vi "oa_Truncate Revolution Indices.vi"(6 "last indices":dbl format="%.2f", 7 "reset? (True)":bool=TRUE, 8 "spectral settings":T2={"window type"=1, "number of lines"=400} {"number of lines" min=2; "window type" items=["None"=0, "Hanning"=1, "Hamming"=2, "Blackman-Harris"=3, "Exact Blackman"=4, "Blackman"=5, "Flat Top"=6, "4 Term B-Harris"=7, "7 Term B-Harris"=8, "Low Sidelobe"=9, "Gaussian"=62]}, 9 "X scale in":cluster{"offset":dbl, "multiplier":dbl} {"multiplier" format="%.2f"; "offset" format="%.2f"}, 10 "rev in":dbl[](array[numeric])=[17.400000000000002, 17.6] format="%.2f", 11 "even-angle signal":cluster{"r0":dbl, "dr":dbl, "Y":dbl[]}={"r0"=0.0, "dr"=1.0, "Y"=[]} {"r0" format="%.2p"; "dr" format="%.2p"; "Y" format="%.2f"}) -> (0 "finished":bool, 1 "scales":T1 {"Y scale"."multiplier" format="%.2f"; "Y scale"."offset" format="%.2f"; "X scale"."multiplier" format="%.2f"; "X scale"."offset" format="%.2f"}, 2 "window indices":dbl[](array[numeric]), 3 "data out":dbl[](array[numeric]) format="%.2f")   [LabVIEW 2017, in "SoundVib_Resampling.lvlib"]
uses:
  <vilib>/addons/Sound and Vibration/Order Analysis/Resample Order Tracking/SoundVib_Resampling.lvlib
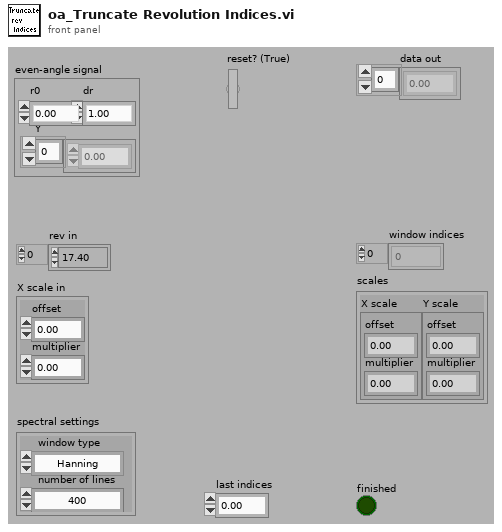
[diagram p1: front panel]
types:
  T1 = cluster{"X scale":cluster{"offset":dbl, "multiplier":dbl}, "Y scale":cluster{"offset":dbl, "multiplier":dbl}}
  T2 = cluster{"window type":u32, "number of lines":i32}
  T3 = cluster{"X scale in":cluster{"offset":dbl, "multiplier":dbl}, cluster{"x/y":dbl, dbl}}
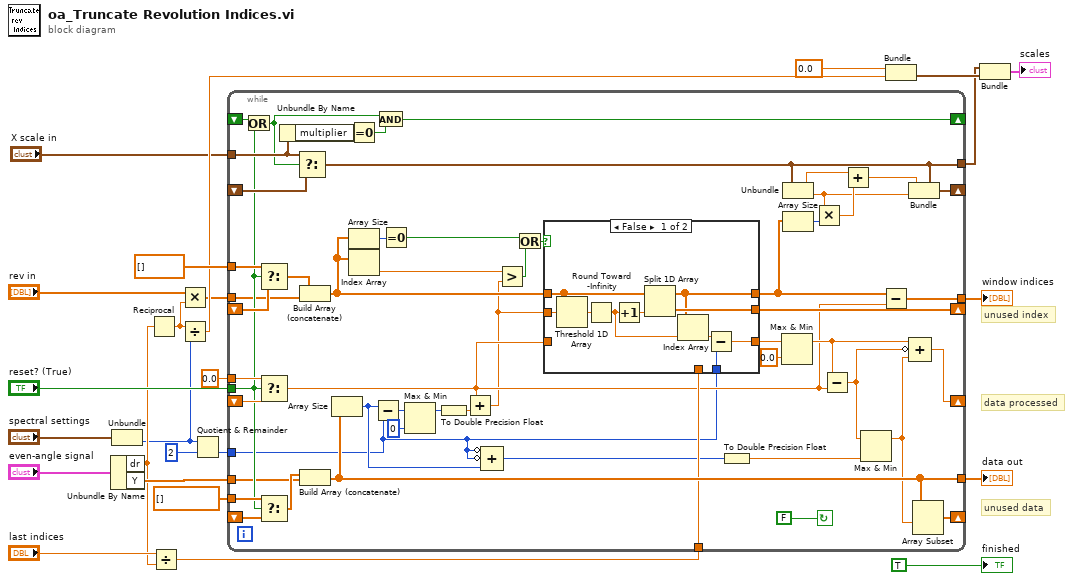
[diagram p0: block diagram]
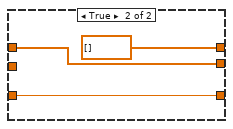
[diagram p2: hidden frame]
diagram:
  # "unused data"
  # "unused index"
  # "data processed"
  n1 = Unbundle By Name("even-angle signal") -> ("dr"=w2:dbl, "Y"=w3:dbl[])
  n2 = Unbundle("spectral settings") -> ("number of lines"=w1:i32)  [unwired: 1 out]
  n3 = Reciprocal(x=w2) -> (1/x=w15:dbl)
  n4 = Divide(x="last indices", y=w2) -> (x/y=w7:dbl)
  n5 = Multiply(x="rev in", y=w15) -> (x*y=w8:dbl[])
  n6 = Divide(x=w15, y=w1) -> (x/y=w14:dbl)
  n7 = Quotient & Remainder(x=w1, y=2) -> (floor(x/y)=w9:i32)  [unwired: 1 out]
  n8 = while {
    shift-right: [w76] -> _
    shift-left: _ -> [w73]
    tunnel: w3 -> [w44]
    shift-right: [w29] -> _
    shift-left: _ -> [w77]
    tunnel: w8 -> [w45]
    tunnel: 0.0 -> [w79]
    shift-right: [w71] -> _
    shift-left: _ -> [w74]
    tunnel: "reset? (True)" -> [w48]
    tunnel: [w70] -> w22
    tunnel: dbl[] [] ("t") -> [w75]
    tunnel: dbl[] [] ("t") -> [w72]
    tunnel: [w67] -> w17
    tunnel: w9 -> [w31]
    tunnel: w7 -> [w60]
    shift-right: [w61] -> _
    shift-left: _ -> [w56]
    tunnel: "X scale in" -> [w53]
    tunnel: [w54] -> w6
    shift-right: [w46] -> _
    shift-left: _ -> [w49]
    stop <- FALSE continue-if-true
    n9 = Or(x=w49, y=w48) -> (x .or. y?=w47:bool)
    n10 = Select(t=w75, s=w48, f=w74) -> (s? t:f=w66:dbl[])
    n11 = Select(t=w79, s=w48, f=w77) -> (s? t:f=w39:dbl)
    n12 = Select(t=w72, s=w48, f=w73) -> (s? t:f=w68:dbl[])
    n13 = Unbundle By Name(w53) -> ("multiplier"=w51:dbl)
    n14 = Select(t=w53, s=w47, f=w56) -> (s? t:f=w54:cluster{"offset":dbl, "multiplier":dbl})
    n15 = Build Array (concatenate)(w66, w45) -> (w38:dbl[])
    n16 = Build Array (concatenate)(w68, w44) -> (w67:dbl[])
    n17 = Array Size(array=w67) -> (size(s)=w32:i32)
    n18 = Equal To 0?(x=w51) -> (x = 0?=w50:bool)
    n19 = Array Size(array=w38) -> (size(s)=w69:i32)
    n20 = Index Array(array=w38) -> (element=w37:dbl)  [unwired: 1 in]
    n21 = Subtract(x=w32, y=w31) -> (x-y=w43:i32)
    n22 = And(x=w47, y=w50) -> (x .and. y?=w46:bool)
    n23 = Equal To 0?(x=w69) -> (x = 0?=w35:bool)
    n24 = Max & Min(x=w43, y=0) -> (max(x,y)=w42:i32)  [unwired: 1 out]
    n25 = To Double Precision Float(number=w42) -> (double precision float=w57:dbl)
    n26 = Add(x=w39, y=w57) -> (x+y=w36:dbl)
    n27 = Compound Arithmetic op=ADD(invert w31, invert w31, w32) -> (w30:i32)
    n28 = Greater?(x=w37, y=w36) -> (0:w34:bool)
    n29 = Or(x=w35, y=w34) -> (x .or. y?=w33:bool)
    n30 = case shown="False" w33 {
      tunnel: w36 -> [w89 _]
      tunnel: [w88 w92] -> w71
      tunnel: w38 -> [w87 w92]
      tunnel: w60 -> [_ _]
      tunnel: [w86 dbl[] []] -> w55
      tunnel: [w85 w90] -> w40
      tunnel: w31 -> [w84 _]
      tunnel: w39 -> [_ w90]
      frame False {
        n31 = Threshold 1D Array(2:w89, 3:w87) -> (0:w83:dbl)  [unwired: 1 in]
        n32 = Round Toward -Infinity(1:w83) -> (0:w82:dbl)
        n33 = Increment(x=w82) -> (x+1=w80:dbl)
        n34 = Split 1D Array(array=w87, index=w80) -> (first subarray=w86:dbl[], second subarray=w88:dbl[])
        n35 = Index Array(array=w86, index=w82) -> (element=w81:dbl)
        n36 = Subtract(x=w81, y=w84) -> (x-y=w85:dbl)
      }
      frame True {
      }
    }
    n37 = To Double Precision Float(number=w30) -> (double precision float=w26:dbl)
    n38 = Max & Min(x=w40, y=0.0) -> (max(x,y)=w58:dbl)  [unwired: 1 out]
    n39 = Unbundle(w54) -> ("offset"=w63:dbl, "multiplier"=w52:dbl)
    n40 = Array Size(array=w55) -> (size(s)=w65:i32)
    n41 = Multiply(x=w52, y=w65) -> (x*y=w64:dbl)
    n42 = Subtract(x=w58, y=w39) -> (x-y=w28:dbl)
    n43 = Add(x=w63, y=w64) -> (x+y=w62:dbl)
    n44 = Max & Min(x=w28, y=w26) -> (max(x,y)=w27:dbl)  [unwired: 1 out]
    n45 = Subtract(x=w55, y=w39) -> (x-y=w70:dbl[])
    n46 = Bundle(cluster=w54, "offset"=w62, "multiplier"=w52) -> (w61:cluster{"offset":dbl, "multiplier":dbl})
    n47 = Compound Arithmetic op=ADD(w58, invert w28, w27) -> (w29:dbl)
    n48 = Array Subset(array=w67, index=w27) -> (w76:dbl[])  [unwired: 1 in]
  }
  "data out" <- w17
  "window indices" <- w22
  n49 = Bundle("x/y"=0.0, w14) -> (w12:cluster{"x/y":dbl, dbl})  [unwired: 1 in]
  n50 = Bundle("X scale in"=w6, w12) -> (→"scales":T3)  [unwired: 1 in]
  "finished" <- TRUE ("finished")
